vi "Set Frame Rate.vi"() -> ()   [LabVIEW 2020]
uses:
  Globals/Status_Frame_Rate_Globals.vi
panel:
  in  "Array 2":dbl[](array[numeric])
  in  "Enum":enum16{"Medium", "High"}(ring)
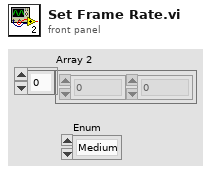
[diagram p1: front panel]
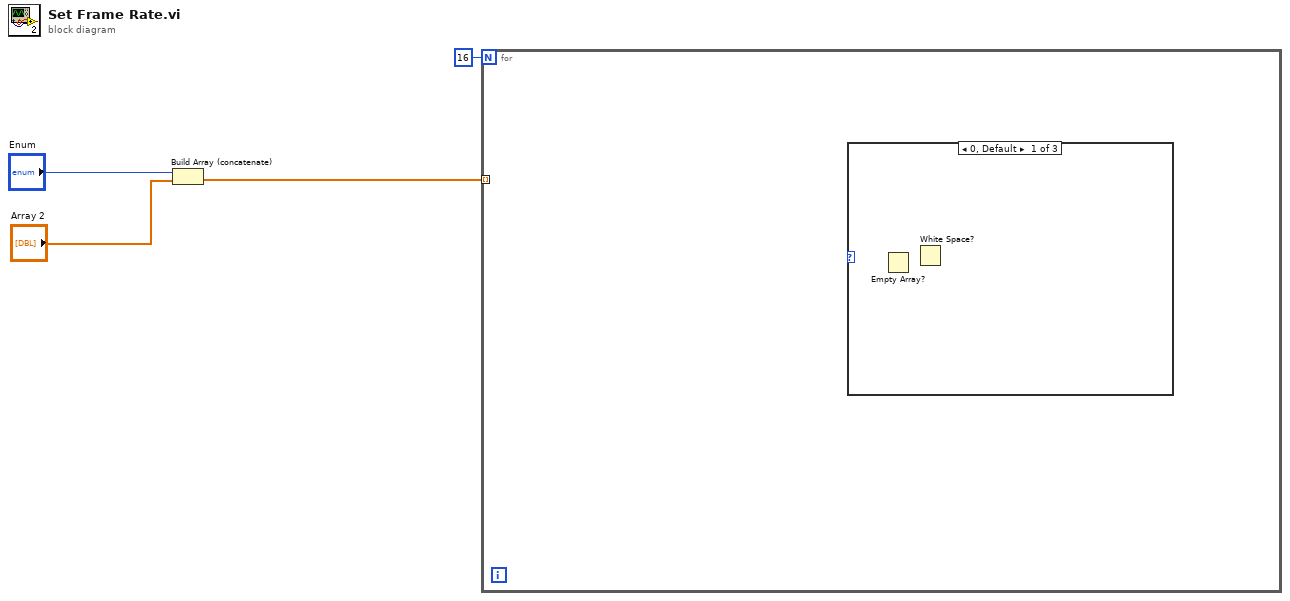
[diagram p0: block diagram]
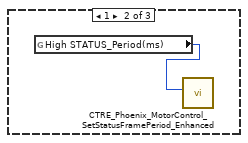
[diagram p2: hidden frame]
diagram:
  n1 = Build Array (concatenate)("Enum", "Array 2") -> (w1:dbl[])
  n2 = for {
    N: 16 -> [_]
    tunnel: w1 -> [_] mode=indexing
    n3 = case shown="0, Default" {
      selector: _ -> [_ _ _]
      frame 0, Default {
        n4 = Empty Array?() -> ()  [unwired: 1 in, 1 out]
        n5 = White Space?() -> ()  [unwired: 1 in, 1 out]
      }
      frame 1 {
        n6 = global read "Status_Frame_Rate_Globals.vi" "High STATUS_Period(ms)"() -> (w5:i32)
        n7 = call <vilib>:"CTRE_Phoenix_MotorControl_SetStatusFramePeriod_Enhanced.vi"("Status Frame"=w5) -> ()  [unwired: 9 in, 2 out]
      }
      frame 2 {
      }
    }
  }
